vi "UsrProfiles-Build window menu.vi"(8 "error in (no error)":errorcluster, 11 "UsrProfiles-Window ref":refnum<k9>) -> (0 "error out":errorcluster, 3 "UsrProfiles-Window ref":refnum<k9>)   [LabVIEW 2020]
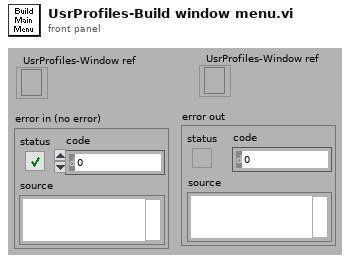
[diagram p1: front panel]
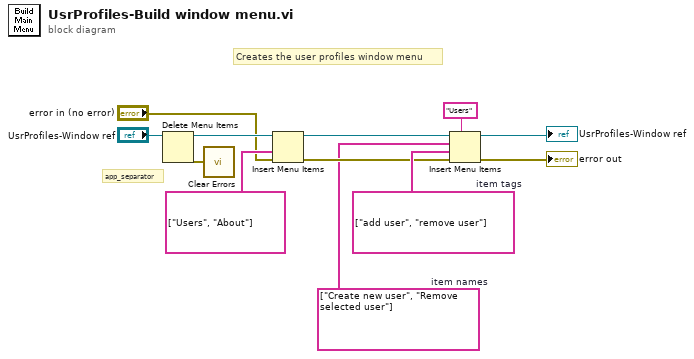
[diagram p0: block diagram]
diagram:
  w3 = string[] ["Create new user", "Remove selected user"]  # item names
  w7 = string[] ["add user", "remove user"]  # item tags
  # "Creates the user profiles window menu"
  # "app_separator"
  n1 = Delete Menu Items(9:"UsrProfiles-Window ref") -> (0:w11:errorcluster, 3:w12:refnum<k9>)  [unwired: 2 in, 1 out]
  n2 = call <vilib>:"Clear Errors.vi"("error in (no error)"=w11) -> ()  [unwired: 5 in, 2 out]
  n3 = Insert Menu Items(6:"error in (no error)", 7:string[] ["Users", "About"] ("item tags"), 9:w12) -> (0:w4:errorcluster, 3:w5:refnum<k9>)  [unwired: 4 out]
  n4 = Insert Menu Items(5:"Users" ("menu tag"), 6:w4, 7:w7, 8:w3, 9:w5) -> (0:→"error out":errorcluster, 3:→"UsrProfiles-Window ref":refnum<k9>)  [unwired: 2 out]
